vi "Read z.vi"(8 "error in (no error)":errorcluster, 11 "Ball in":refnum<class "Ball.lvclass">) -> (0 "error out":errorcluster, 2 "z":dbl, 3 "Ball out":refnum<class "Ball.lvclass">)   [LabVIEW 2023, in "Ball.lvclass"]
uses:
  Ball.lvclass
  Ball.lvclass/Ball.ctl
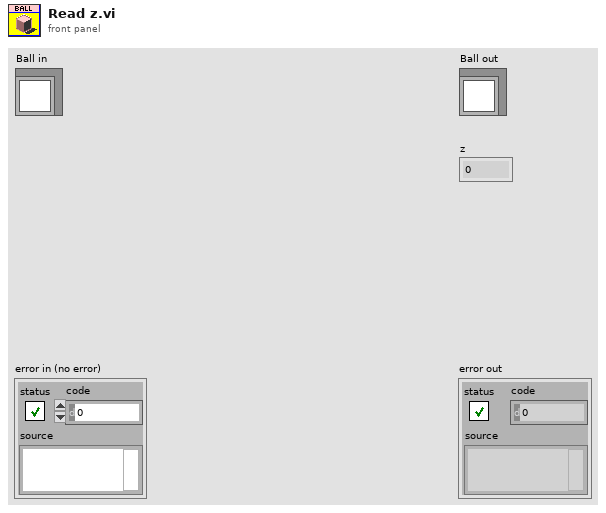
[diagram p1: front panel]
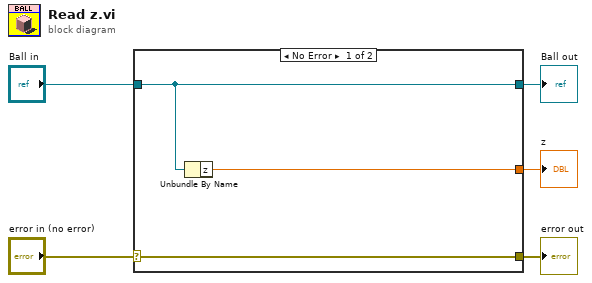
[diagram p0: block diagram]
diagram:
  n1 = case shown="No Error" "error in (no error)" {
    selector: "error in (no error)" -> [w8 w9]
    tunnel: [w8 w9] -> w4
    tunnel: [w7 w10] -> w2
    tunnel: "Ball in" -> [w7 w10]
    tunnel: [w6 _] -> w1
    frame No Error {
      n2 = Unbundle By Name(w7) -> ("z"=w6:dbl)
    }
    frame Error {
    }
  }
  "error out" <- w4
  "Ball out" <- w2
  "z" <- w1
